vi "Initialize Popup.vi"(8 "error in (no error)":errorcluster, 9 "Size":T2, 10 "Screen Coordinates":T1, 11 "Numeric Data Type in":refnum<class "Numeric Data Type.lvclass">) -> (0 "error out":errorcluster, 2 "Dialog":refnum<class "Dialog.lvclass">, 3 "Numeric Data Type out":refnum<class "Numeric Data Type.lvclass">)   [LabVIEW 2018, in "Numeric Data Type.lvclass"]
uses:
  Numeric Data Type.lvclass
  <vilib>/MGI/Panel Manager/Panel/Panel/Window/Dialog/Dialog.lvclass
  <vilib>/Utility/miscctls.llb/LVBoundsTypeDef.ctl
  <vilib>/Utility/miscctls.llb/LVPointTypeDef.ctl
  Numeric Data Type.lvclass/Numeric Data Type.ctl
  <vilib>/MGI/Panel Manager/Panel/Panel/Window/Dialog/Behavior.ctl
  <vilib>/MGI/Panel Manager/Panel/Window Position/Reference Position/Size/Absolute Size/Absolute Size.lvclass/Absolute Size.ctl
  <vilib>/MGI/Panel Manager/Panel/Window Position/Reference Position/Offset/Absolute Offset/Absolute Offset.lvclass/Absolute Offset.ctl
  <vilib>/MGI/Panel Manager/Panel/Window Position/Reference Position/Size/Absolute Size/Absolute Size.vi
  <vilib>/MGI/Panel Manager/Panel/Window Position/Reference Position/Offset/Absolute Offset/Absolute Offset.vi
  <vilib>/MGI/Panel Manager/Panel/Window Position/Reference Position/Size/Absolute Size/Absolute Size.lvclass
  C:/Program Files (x86)/National Instruments/LabVIEW 2018/vi.lib/MGI/Panel Manager/Panel/Window Position/Reference Position/Size/Size.lvclass
  <vilib>/MGI/Panel Manager/Panel/Window Position/Reference Position/Offset/Absolute Offset/Absolute Offset.lvclass
  C:/Program Files (x86)/National Instruments/LabVIEW 2018/vi.lib/MGI/Panel Manager/Panel/Window Position/Reference Position/Offset/Offset.lvclass
  <vilib>/MGI/Panel Manager/Panel/Window Position/Reference Position/Ref Display/Ref Display.lvclass
  C:/Program Files (x86)/National Instruments/LabVIEW 2018/vi.lib/MGI/Panel Manager/Panel/Window Position/Window Position.lvclass
  <vilib>/MGI/Panel Manager/Panel/Window Position/Reference Position/Ref Display/Ref Display.vi
  <vilib>/MGI/Panel Manager/Panel/Panel/Window/Dialog/Dialog.vi
  <vilib>/MGI/Panel Manager/Panel/Panel.lvlib
  C:/Program Files (x86)/National Instruments/LabVIEW 2018/vi.lib/MGI/Panel Manager/Panel/Window Position/Reference Position/Reference Position.lvclass
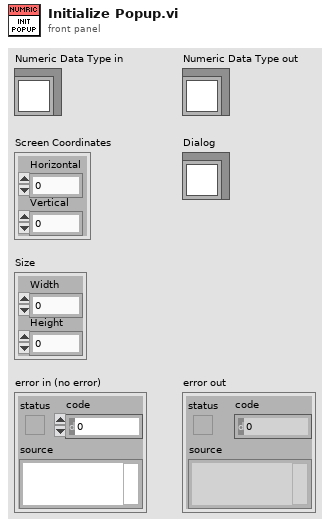
[diagram p1: front panel]
types:
  T1 = typedef "LVPointTypeDef.ctl" = cluster{"Horizontal":i16, "Vertical":i16}
  T2 = typedef "LVBoundsTypeDef.ctl" = cluster{"Width":u32, "Height":u32}
  T3 = typedef "Panel.lvlib/Dialog.lvclass/Behavior.ctl" = enum32{"Floating", "Floating/Auto-Hide", "Modal"}
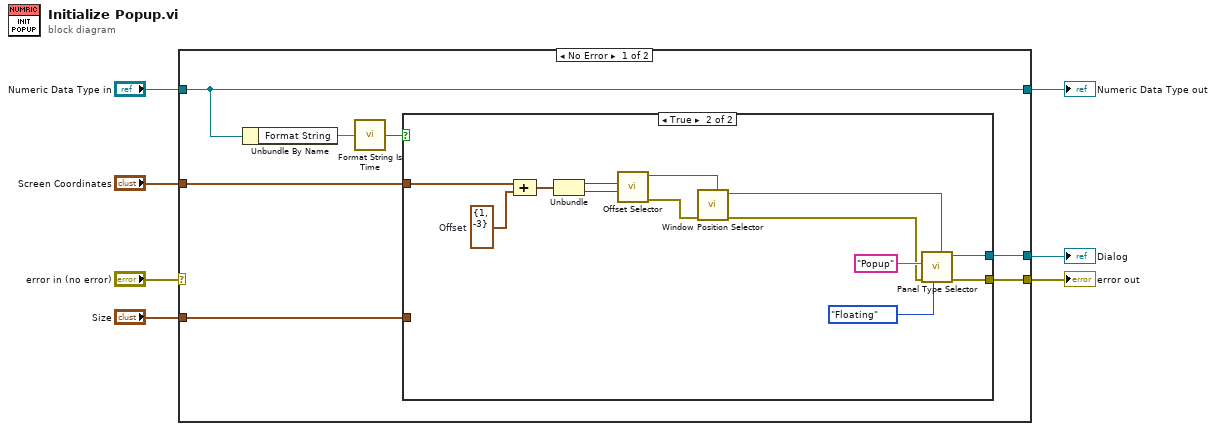
[diagram p0: block diagram]
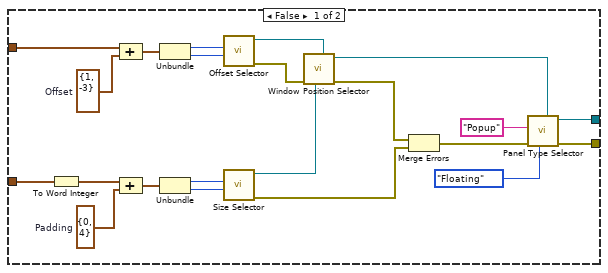
[diagram p2: hidden frame]
diagram:
  n1 = case shown="No Error" "error in (no error)" {
    selector: "error in (no error)" -> [_ w51]
    tunnel: [w13 w51] -> w1
    tunnel: [w10 w50] -> w6
    tunnel: "Numeric Data Type in" -> [w10 w50]
    tunnel: [w14 _] -> w2
    tunnel: "Screen Coordinates" -> [w12 _]
    tunnel: "Size" -> [w11 _]
    frame No Error {
      n2 = Unbundle By Name(w10) -> ("Format String"=w9:string)
      n3 = call "Format String Is Time.vi"("Format String"=w9) -> ("Time?"=w8:bool)
      n4 = case shown="True" w8 {
        tunnel: [w22 w41] -> w14
        tunnel: [w17 w38] -> w13
        tunnel: w12 -> [w16 w37]
        tunnel: w11 -> [w15 _]
        frame False {
          w35 = cluster{"Width":i16, "Height":i16} {"Width"=1, "Height"=-3}  # Offset
          w31 = cluster{"Width":i16, "Height":i16} {"Width"=0, "Height"=4}  # Padding
          n5 = To Word Integer(number=w15) -> (16bit integer=w29:cluster{"Width":i16, "Height":i16})
          n6 = Compound Arithmetic op=ADD(w16, w35) -> (w34:T1)
          n7 = Compound Arithmetic op=ADD(w29, w31) -> (w30:cluster{"Width":i16, "Height":i16})
          n8 = Unbundle(w34) -> ("Horizontal"=w32:i16, "Vertical"=w33:i16)
          n9 = Unbundle(w30) -> ("Width"=w27:i16, "Height"=w28:i16)
          n10 = call-poly <vilib>:"Offset Selector.vi"("Vertical"=w33, "Horizontal"=w32) -> ("Error Out"=w21:errorcluster, "Absolute Offset Out"=w26:refnum<class "Absolute Offset.lvclass">)  [unwired: 8 in]
          n11 = call-poly <vilib>:"Size Selector.vi"("Height"=w28, "Width"=w27) -> ("Error Out"=w18:errorcluster, "Absolute Size out"=w25:refnum<class "Absolute Size.lvclass">)  [unwired: 8 in]
          n12 = call-poly <vilib>:"Window Position Selector.vi"("Offset"=w26, "Size"=w25, "Error In"=w21) -> ("Error Out"=w19:errorcluster, "Ref Display out"=w24:refnum<class "Ref Display.lvclass">)  [unwired: 7 in]
          n13 = Merge Errors(w19, w18) -> (w20:errorcluster)
          n14 = call-poly <vilib>:"Panel Type Selector.vi"("Window Position (Center in Top Level)"=w24, "Behavior (Modal)"=Behavior."Floating", "Error In"=w20, "Default Title"="Popup") -> ("Error Out"=w17:errorcluster, "Dialog out"=w22:refnum<class "Dialog.lvclass">)  [unwired: 6 in]
        }
        frame True {
          w48 = cluster{"Width":i16, "Height":i16} {"Width"=1, "Height"=-3}  # Offset
          n15 = Compound Arithmetic op=ADD(w37, w48) -> (w47:T1)
          n16 = Unbundle(w47) -> ("Horizontal"=w45:i16, "Vertical"=w46:i16)
          n17 = call-poly <vilib>:"Offset Selector.vi"("Vertical"=w46, "Horizontal"=w45) -> ("Error Out"=w40:errorcluster, "Absolute Offset Out"=w44:refnum<class "Absolute Offset.lvclass">)  [unwired: 8 in]
          n18 = call-poly <vilib>:"Window Position Selector.vi"("Offset"=w44, "Error In"=w40) -> ("Error Out"=w39:errorcluster, "Ref Display out"=w43:refnum<class "Ref Display.lvclass">)  [unwired: 8 in]
          n19 = call-poly <vilib>:"Panel Type Selector.vi"("Window Position (Center in Top Level)"=w43, "Behavior (Modal)"=Behavior."Floating", "Error In"=w39, "Default Title"="Popup") -> ("Error Out"=w38:errorcluster, "Dialog out"=w41:refnum<class "Dialog.lvclass">)  [unwired: 6 in]
        }
      }
    }
    frame Error {
    }
  }
  "error out" <- w1
  "Numeric Data Type out" <- w6
  "Dialog" <- w2
